vi "UTILITY Elapsed Time General Info.vi"(5 "Add Elapsed Time (hrs)":bool, 6 "precision (6)":i16=6, 7 "Add Software Elapsed Time":bool, 8 "Error In":errorcluster, 10 "Software Elapsed Time":dbl format="%<%H:%M:%S>t", 11 "Elapsed Time (sec)":dbl) -> (0 "Error Out":errorcluster, 1 "Main Loop Rate":dbl format="%0.2f", 2 "Total Array":string[][](array[string]), 3 "Elapsed Time":dbl, 4 "Main Start":dbl format="%.2f")   [LabVIEW 2020]
uses:
  <vilib>/ptbypt/NI_PtbyPt.lvlib
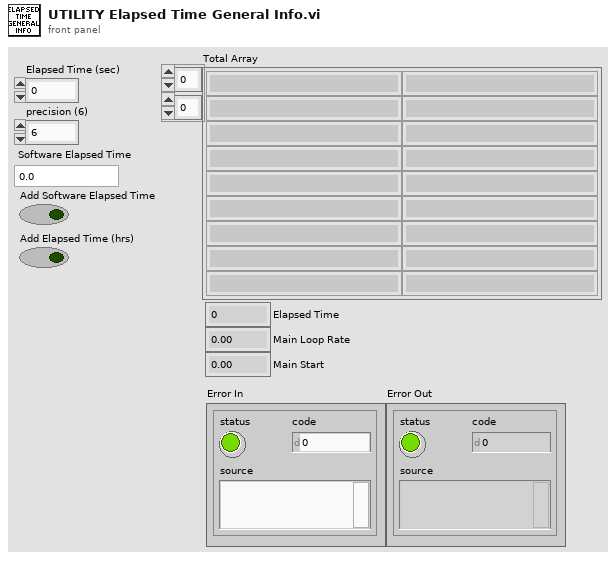
[diagram p1: front panel]
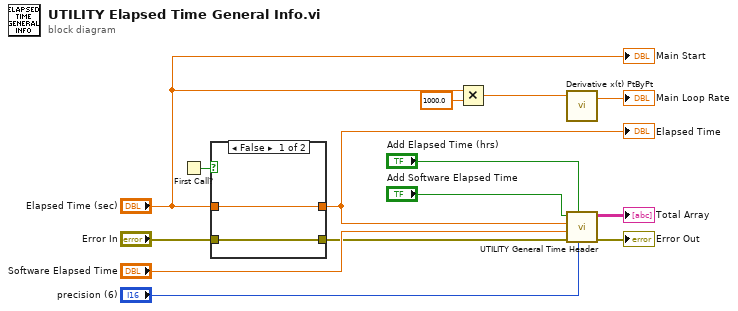
[diagram p0: block diagram]
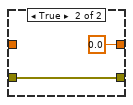
[diagram p2: hidden frame]
diagram:
  n1 = First Call?() -> (First Call?: T/F=w14:bool)
  n2 = case shown="False" w14 {
    tunnel: [w16 0.0 ("Start")] -> w12
    tunnel: "Elapsed Time (sec)" -> [w16 _]
    tunnel: "Error In" -> [w15 w17]
    tunnel: [w15 w17] -> w2
    frame False {
    }
    frame True {
    }
  }
  "Elapsed Time" <- w12
  n3 = Multiply(x="Elapsed Time (sec)", y=1000.0) -> (x*y=w10:dbl)
  n4 = call <vilib>:"Derivative x(t) PtByPt.vi"("x"=w10) -> ("dx/dt"=→"Main Loop Rate":dbl)  [unwired: 3 in, 1 out]
  n5 = call "UTILITY General Time Header.vi"("precision (6)"="precision (6)", "Add Elapsed Time (hrs)"="Add Elapsed Time (hrs)", "Error In"=w2, "Software Elapsed Time"="Software Elapsed Time", "Elapsed Time"=w12, "Add Software Elapsed Time"="Add Software Elapsed Time") -> ("Error Out"=→"Error Out":errorcluster, "Total Array"=→"Total Array":string[][])  [unwired: 4 in]
  "Main Start" <- "Elapsed Time (sec)"
